vi "DriveEncoderRate.vi"(10 "EncoderRate":dbl) -> (2 "RateOut":dbl)   [LabVIEW 2013]
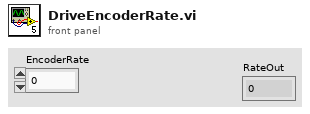
[diagram p1: front panel]
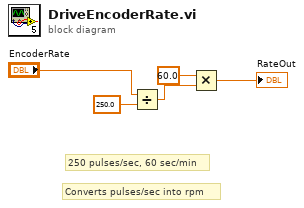
[diagram p0: block diagram]
diagram:
  # "Converts pulses/sec into rpm"
  # "250 pulses/sec, 60 sec/min"
  n1 = Divide(x="EncoderRate", y=250.0) -> (x/y=w3:dbl)
  n2 = Multiply(x=60.0, y=w3) -> (x*y=→"RateOut":dbl)
